vi "ftruncate.vi"(8 "error in (no error)":errorcluster, 10 "size (bytes)":u32, 11 "file descriptor":i32) -> (0 "error out":errorcluster, 2 "size (bytes)":u32, 3 "file descriptor":i32)   [LabVIEW 2013, in "Shared Memory.lvlib" / "Shared Memory.lvclass"]
doc: "Wrapper VI for Linux function ftruncate()."
uses:
  Shared Memory.lvclass
  Controls/functions.ctl
  <vilib>/NI/NI Linux RT Errno/Linux Errno.lvlib
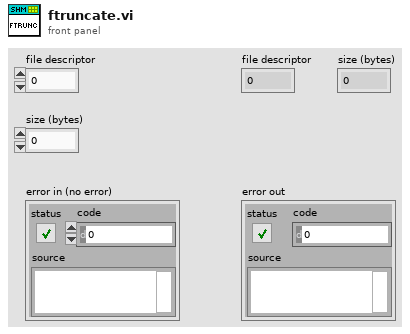
[diagram p1: front panel]
types:
  T1 = typedef "Shared Memory.lvlib/Shared Memory.lvclass/functions.ctl" = enum16{"unspecified", "shm_open", "ftruncate", "mmap", "munmap", "close", "shm_unlink", "fstat"}
  T2 = typedef "Linux Errno.lvlib/errno.ctl" = enum16{"NO ERROR", "EPERM", "ENOENT", "ESRCH", "EINTR", "EIO", "ENXIO", "E2BIG", "ENOEXEC", "EBADF", "ECHILD", "EAGAIN", "ENOMEM", "EACCES", "EFAULT", "ENOTBLK", "EBUSY", "EEXIST", "EXDEV", "ENODEV", "ENOTDIR", "EISDIR", "EINVAL", "ENFILE", "EMFILE", "ENOTTY", "ETXTBSY", "EFBIG", "ENOSPC", "ESPIPE", "EROFS", "EMLINK", "EPIPE", "EDOM", "ERANGE", "EDADLK", "ENAMETOOLONG", "ENOLCK", "ENOSYS", "ENOTEMPTY", "ELOOP", "EWOULDBLOCK", "ENOMSG", "EIDRM", "ECHRNG", "EL2NSYNC", "EL3HLT", "EL3RST", "ELNRNG", "EUNATCH", "ENOCSI", "EL2HLT", "EBADE", "EBADR", "EXFULL", "ENOANO", "EBADRQC", "EBADSLT", "EDEADLOCK", "EBFONT", "ENOSTR", "ENODATA", "ETIME", "ENOSR", "ENONET", "ENOPKG", "EREMOTE", "ENOLINK", "EADV", "ESRMNT", "ECOMM", "EPROTO", "EMULTIHOP", "EDOTDOT", "EBADMSG", "EOVERFLOW", "ENOTUNIQ", "EBADFD", "EREMCHG", "ELIBACC", "ELIBBAD", "ELIBSCN", "ELIBMAX", "ELIBEXEC", "ELISEQ", "ERESTART", "ESTRPIPE", "EUSERS", "ENOTSOCK", "EDESTADDRREQ", "EMSGSIZE", "EPROTOTYPE", "ENOPROTOOPT", "EPROTONOSUPPORT", "ESOCKTNOSUPPORT", "EOPNOTSUPP", "EPFNOSUPPORT", "EAFNOSUPPORT", "EADDRINUSE", "EADDRNOTAVAIL", "ENETDOWN", "ENETUNREACH", "ENETRESET", "ECONNABORTED", "ECONNRESET", "ENOBUFS", "EISCONN", "ENOTCONN", "ESHUTDOWN", "ETOOMANYREFS", "ETIMEDOUT", "ECONNREFUSED", "EHOSTDOWN", "EHOSTUNREACH", "EALREADY", "EINPROGRESS", "ESTALE", "EUCLEAN", "ENOTNAM", "ENAVAIL", "EISNAM", "EREMOTEIO", "EDQUOT", "ENOMEDIUM", "EMEDIUMTYPE", "ECANCELED", "ENOKEY", "EKEYEXPIRED", "EKEYREVOKED", "EKEYREJECTED", "EOWNERDEAD", "ENOTRECOVERABLE", "ERFKILL", "EHWPOISON", "UNDEFINED"}
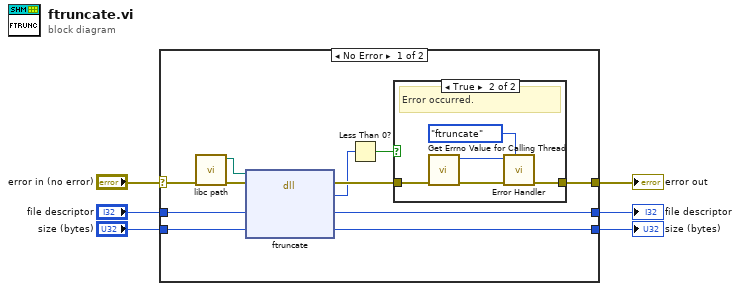
[diagram p0: block diagram]
diagram:
  n1 = case shown="No Error" "error in (no error)" {
    selector: "error in (no error)" -> [w14 w25]
    tunnel: "file descriptor" -> [w17 w24]
    tunnel: "size (bytes)" -> [w16 _]
    tunnel: [w9 w25] -> w4
    tunnel: [w15 w24] -> w3
    tunnel: [w13 _] -> w1
    frame No Error {
      n2 = call "libc path.vi"("error in (no error)"=w14) -> ("error out"=w12:errorcluster, "path to libc"=w11:path)  [unwired: 9 in]
      n3 = dll-call lib="?" fn="ftruncate"(path in=w11, error in=w12, "fd"=w17, "length"=w16) -> (error out=w10:errorcluster, "status"=w7:i32, "fd"=w15:i32, "length"=w13:u32)  [unwired: 1 in, 1 out]
      n4 = Less Than 0?(x=w7) -> (x < 0?=w8:bool)
      n5 = case shown="True" w8 {
        tunnel: w10 -> [w18 w23]
        tunnel: [w18 w20] -> w9
        frame False {
          # "No error."
        }
        frame True {
          # "Error occurred."
          n6 = call <vilib>:"Get Errno Value for Calling Thread.vi"("error in (no error)"=w23) -> ("error out"=w21:errorcluster, "errno"=w19:T2)  [unwired: 9 in]
          n7 = call "Error Handler.vi"("function"=functions."ftruncate", "error in (no error)"=w21, "errno"=w19) -> ("error out"=w20:errorcluster)  [unwired: 8 in]
        }
      }
    }
    frame Error {
    }
  }
  "error out" <- w4
  "file descriptor" <- w3
  "size (bytes)" <- w1
